vi "Wheel Speed Sensors.vi"() -> (3 "ticks/count":u32)   [LabVIEW 2011]
uses:
  <vilib>/rvi/eio/common/nirviEmuTemplateMethod_errors.vi
  <vilib>/eio/EIONode/EIONode.xnode
panel:
  in  "stop":bool
  out "ticks/count 4":u32
  out "ticks/count 3":u32
  out "ticks/count 2":u32
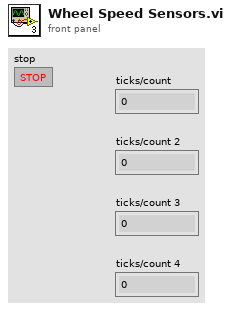
[diagram p1: front panel]
types:
  T1 = enum16{"Wheel Speed 1", "Wheel Speed 2", "Wheel Speed 3", "Wheel Speed 4"}
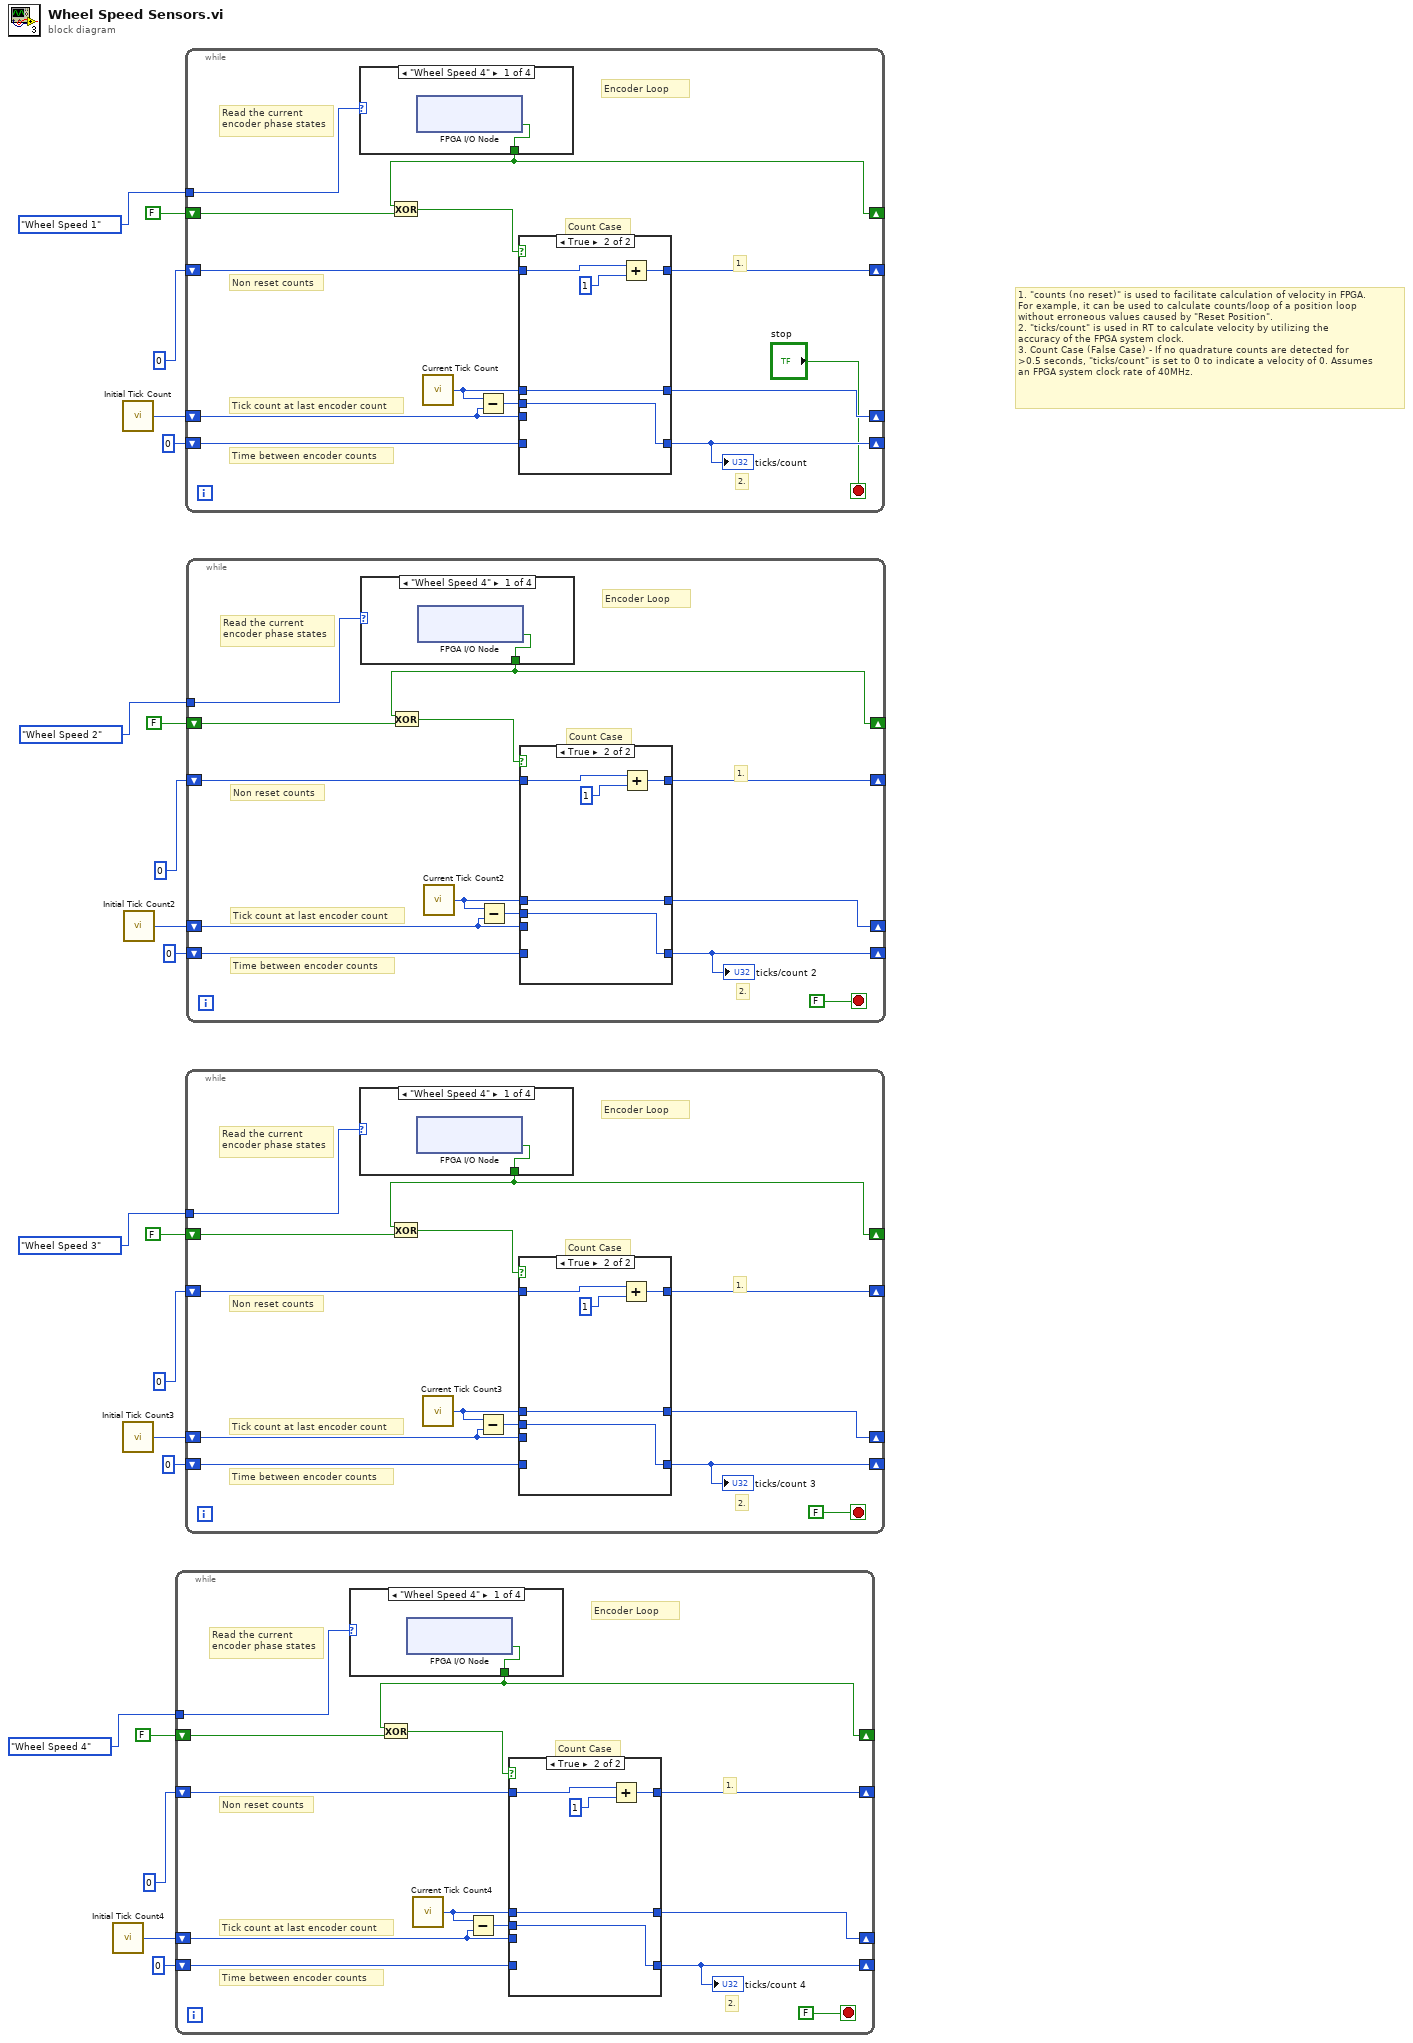
[diagram p0: block diagram]
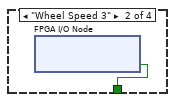
[diagram p2: hidden frame]
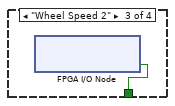
[diagram p3: hidden frame]
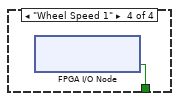
[diagram p4: hidden frame]
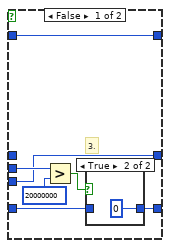
[diagram p5: hidden frame]
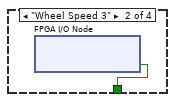
[diagram p7: hidden frame]
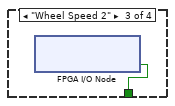
[diagram p8: hidden frame]
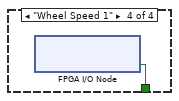
[diagram p9: hidden frame]
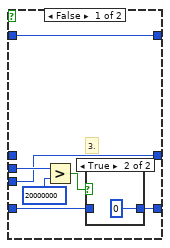
[diagram p10: hidden frame]
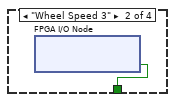
[diagram p12: hidden frame]
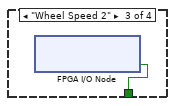
[diagram p13: hidden frame]
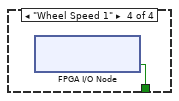
[diagram p14: hidden frame]
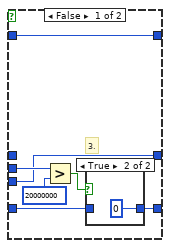
[diagram p15: hidden frame]
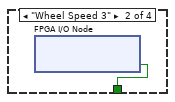
[diagram p17: hidden frame]
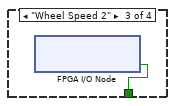
[diagram p18: hidden frame]
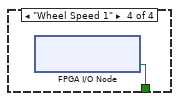
[diagram p19: hidden frame]
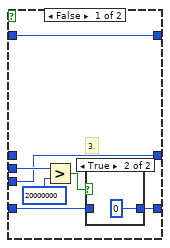
[diagram p20: hidden frame]
diagram:
  # "1. \"counts (no reset)\" is used to facilitate calculation of velocity in FPGA.\nFor example, it can be used to calculate counts/loop of a position loop\nwithout erroneous values caused by \"Reset Position\". \n2. \"ticks/count\" is used in RT to calculate velocity by utilizing the\naccuracy of the FPGA system clock.\n3. Count Case (False Case) - If no quadrature counts are detected for\n>0.5 seconds, \"ticks/count\" is set to 0 to indicate a velocity of 0. Assumes\nan FPGA system clock rate of 40MHz."
  n1 = call "Initial Tick Count4"() -> ("Tick Count(Ticks)"=w3:u32)
  n2 = call "Initial Tick Count"() -> ("Tick Count(Ticks)"=w18:u32)
  n3 = call "Initial Tick Count3"() -> ("Tick Count(Ticks)"=w8:u32)
  n4 = call "Initial Tick Count2"() -> ("Tick Count(Ticks)"=w13:u32)
  n5 = while {
    shift-right: [w21] -> _
    shift-left: FALSE ("Encoder Phase A") -> [w33]
    shift-right: [w32] -> _
    shift-left: w3 -> [w26]
    shift-right: [w31] -> _
    shift-left: u32 0 -> [w30]
    shift-right: [w27] -> _
    shift-left: 0 ("Reset Position Value") -> [w28]
    tunnel: T1."Wheel Speed 4" ("Sensor Number") -> [w22]
    stop <- FALSE stop-if-true
    # "Encoder Loop"
    # "Count Case"
    # "2."
    # "1."
    # "Read the current\nencoder phase states"
    # "Non reset counts"
    # "Time between encoder counts"
    # "Tick count at last encoder count"
    n6 = case shown="\"Wheel Speed 4\"" w22 {
      tunnel: [w34 w35 w36 w37] -> w21
      frame "Wheel Speed 4" {
        n7 = xnode "FPGA I/O Node"() -> ("Mod1/DIO4"=w34:bool)  [unwired: 1 in, 1 out]
      }
      frame "Wheel Speed 3" {
        n8 = xnode "FPGA I/O Node"() -> ("Mod1/DIO2"=w35:bool)  [unwired: 1 in, 1 out]
      }
      frame "Wheel Speed 2" {
        n9 = xnode "FPGA I/O Node"() -> ("Mod1/DIO1"=w36:bool)  [unwired: 1 in, 1 out]
      }
      frame "Wheel Speed 1" {
        n10 = xnode "FPGA I/O Node"() -> ("Mod1/DIO0"=w37:bool)  [unwired: 1 in, 1 out]
      }
    }
    n11 = Exclusive Or(1:w33, 2:w21) -> (0:w23:bool)
    n12 = call "Current Tick Count4"() -> ("Tick Count(Ticks)"=w24:u32)
    n13 = Subtract(x=w24, y=w26) -> (x-y=w25:u32)
    n14 = case shown="True" w23 {
      tunnel: [w38 w49] -> w32
      tunnel: w26 -> [w38 _]
      tunnel: [w41 w48] -> w31
      tunnel: w30 -> [w40 _]
      tunnel: [w44 w51] -> w27
      tunnel: w28 -> [w44 w50]
      tunnel: w25 -> [w39 w48]
      tunnel: w24 -> [_ w49]
      frame False {
        # "3."
        n15 = Greater?(x=w39, y=20000000 ("x")) -> (0:w42:bool)
        n16 = case shown="True" w42 {
          tunnel: [w45 u32 0] -> w41
          tunnel: w40 -> [w45 _]
          frame False {
          }
          frame True {
          }
        }
      }
      frame True {
        n17 = Add(x=w50, y=1 ("16 bit")) -> (x+y=w51:i32)
      }
    }
    "ticks/count 4" <- w31
  }
  n18 = while {
    shift-right: [w53] -> _
    shift-left: FALSE ("Encoder Phase A") -> [w64]
    shift-right: [w63] -> _
    shift-left: w18 -> [w58]
    shift-right: [w62] -> _
    shift-left: u32 0 -> [w61]
    shift-right: [w59] -> _
    shift-left: 0 ("Reset Position Value") -> [w60]
    tunnel: T1."Wheel Speed 1" ("Sensor Number") -> [w54]
    stop <- "stop" stop-if-true
    # "Encoder Loop"
    # "Count Case"
    # "2."
    # "1."
    # "Read the current\nencoder phase states"
    # "Non reset counts"
    # "Time between encoder counts"
    # "Tick count at last encoder count"
    n19 = case shown="\"Wheel Speed 4\"" w54 {
      tunnel: [w65 w66 w67 w68] -> w53
      frame "Wheel Speed 4" {
        n20 = xnode "FPGA I/O Node"() -> ("Mod1/DIO4"=w65:bool)  [unwired: 1 in, 1 out]
      }
      frame "Wheel Speed 3" {
        n21 = xnode "FPGA I/O Node"() -> ("Mod1/DIO2"=w66:bool)  [unwired: 1 in, 1 out]
      }
      frame "Wheel Speed 2" {
        n22 = xnode "FPGA I/O Node"() -> ("Mod1/DIO1"=w67:bool)  [unwired: 1 in, 1 out]
      }
      frame "Wheel Speed 1" {
        n23 = xnode "FPGA I/O Node"() -> ("Mod1/DIO0"=w68:bool)  [unwired: 1 in, 1 out]
      }
    }
    n24 = Exclusive Or(1:w64, 2:w53) -> (0:w55:bool)
    n25 = call "Current Tick Count"() -> ("Tick Count(Ticks)"=w56:u32)
    n26 = Subtract(x=w56, y=w58) -> (x-y=w57:u32)
    n27 = case shown="True" w55 {
      tunnel: [w69 w80] -> w63
      tunnel: w58 -> [w69 _]
      tunnel: [w72 w79] -> w62
      tunnel: w61 -> [w71 _]
      tunnel: [w75 w82] -> w59
      tunnel: w60 -> [w75 w81]
      tunnel: w57 -> [w70 w79]
      tunnel: w56 -> [_ w80]
      frame False {
        # "3."
        n28 = Greater?(x=w70, y=20000000 ("x")) -> (0:w73:bool)
        n29 = case shown="True" w73 {
          tunnel: [w76 u32 0] -> w72
          tunnel: w71 -> [w76 _]
          frame False {
          }
          frame True {
          }
        }
      }
      frame True {
        n30 = Add(x=w81, y=1 ("16 bit")) -> (x+y=w82:i32)
      }
    }
    "ticks/count" <- w62
  }
  n31 = while {
    shift-right: [w83] -> _
    shift-left: FALSE ("Encoder Phase A") -> [w95]
    shift-right: [w94] -> _
    shift-left: w8 -> [w88]
    shift-right: [w93] -> _
    shift-left: u32 0 -> [w92]
    shift-right: [w89] -> _
    shift-left: 0 ("Reset Position Value") -> [w90]
    tunnel: T1."Wheel Speed 3" ("Sensor Number") -> [w84]
    stop <- FALSE stop-if-true
    # "Encoder Loop"
    # "Count Case"
    # "2."
    # "1."
    # "Read the current\nencoder phase states"
    # "Non reset counts"
    # "Time between encoder counts"
    # "Tick count at last encoder count"
    n32 = case shown="\"Wheel Speed 4\"" w84 {
      tunnel: [w96 w97 w98 w99] -> w83
      frame "Wheel Speed 4" {
        n33 = xnode "FPGA I/O Node"() -> ("Mod1/DIO4"=w96:bool)  [unwired: 1 in, 1 out]
      }
      frame "Wheel Speed 3" {
        n34 = xnode "FPGA I/O Node"() -> ("Mod1/DIO2"=w97:bool)  [unwired: 1 in, 1 out]
      }
      frame "Wheel Speed 2" {
        n35 = xnode "FPGA I/O Node"() -> ("Mod1/DIO1"=w98:bool)  [unwired: 1 in, 1 out]
      }
      frame "Wheel Speed 1" {
        n36 = xnode "FPGA I/O Node"() -> ("Mod1/DIO0"=w99:bool)  [unwired: 1 in, 1 out]
      }
    }
    n37 = Exclusive Or(1:w95, 2:w83) -> (0:w85:bool)
    n38 = call "Current Tick Count3"() -> ("Tick Count(Ticks)"=w86:u32)
    n39 = Subtract(x=w86, y=w88) -> (x-y=w87:u32)
    n40 = case shown="True" w85 {
      tunnel: [w100 w111] -> w94
      tunnel: w88 -> [w100 _]
      tunnel: [w103 w110] -> w93
      tunnel: w92 -> [w102 _]
      tunnel: [w106 w113] -> w89
      tunnel: w90 -> [w106 w112]
      tunnel: w87 -> [w101 w110]
      tunnel: w86 -> [_ w111]
      frame False {
        # "3."
        n41 = Greater?(x=w101, y=20000000 ("x")) -> (0:w104:bool)
        n42 = case shown="True" w104 {
          tunnel: [w107 u32 0] -> w103
          tunnel: w102 -> [w107 _]
          frame False {
          }
          frame True {
          }
        }
      }
      frame True {
        n43 = Add(x=w112, y=1 ("16 bit")) -> (x+y=w113:i32)
      }
    }
    "ticks/count 3" <- w93
  }
  n44 = while {
    shift-right: [w114] -> _
    shift-left: FALSE ("Encoder Phase A") -> [w126]
    shift-right: [w125] -> _
    shift-left: w13 -> [w119]
    shift-right: [w124] -> _
    shift-left: u32 0 -> [w123]
    shift-right: [w120] -> _
    shift-left: 0 ("Reset Position Value") -> [w121]
    tunnel: T1."Wheel Speed 2" ("Sensor Number") -> [w115]
    stop <- FALSE stop-if-true
    # "Encoder Loop"
    # "Count Case"
    # "2."
    # "1."
    # "Read the current\nencoder phase states"
    # "Non reset counts"
    # "Time between encoder counts"
    # "Tick count at last encoder count"
    n45 = case shown="\"Wheel Speed 4\"" w115 {
      tunnel: [w127 w128 w129 w130] -> w114
      frame "Wheel Speed 4" {
        n46 = xnode "FPGA I/O Node"() -> ("Mod1/DIO4"=w127:bool)  [unwired: 1 in, 1 out]
      }
      frame "Wheel Speed 3" {
        n47 = xnode "FPGA I/O Node"() -> ("Mod1/DIO2"=w128:bool)  [unwired: 1 in, 1 out]
      }
      frame "Wheel Speed 2" {
        n48 = xnode "FPGA I/O Node"() -> ("Mod1/DIO1"=w129:bool)  [unwired: 1 in, 1 out]
      }
      frame "Wheel Speed 1" {
        n49 = xnode "FPGA I/O Node"() -> ("Mod1/DIO0"=w130:bool)  [unwired: 1 in, 1 out]
      }
    }
    n50 = Exclusive Or(1:w126, 2:w114) -> (0:w116:bool)
    n51 = call "Current Tick Count2"() -> ("Tick Count(Ticks)"=w117:u32)
    n52 = Subtract(x=w117, y=w119) -> (x-y=w118:u32)
    n53 = case shown="True" w116 {
      tunnel: [w131 w142] -> w125
      tunnel: w119 -> [w131 _]
      tunnel: [w134 w141] -> w124
      tunnel: w123 -> [w133 _]
      tunnel: [w137 w144] -> w120
      tunnel: w121 -> [w137 w143]
      tunnel: w118 -> [w132 w141]
      tunnel: w117 -> [_ w142]
      frame False {
        # "3."
        n54 = Greater?(x=w132, y=20000000 ("x")) -> (0:w135:bool)
        n55 = case shown="True" w135 {
          tunnel: [w138 u32 0] -> w134
          tunnel: w133 -> [w138 _]
          frame False {
          }
          frame True {
          }
        }
      }
      frame True {
        n56 = Add(x=w143, y=1 ("16 bit")) -> (x+y=w144:i32)
      }
    }
    "ticks/count 2" <- w124
  }
